vi "4060_outputs.vi"(0 "Address":T1, 3 "Value to Output":dbl format="%.2f", 4 "Channel Name":string) -> (5 "Comment":string, 6 "Reading":dbl format="%.3f")   [LabVIEW 2018]
uses:
  ADAM Client/Sub VIs/ADAM Controls/Address.ctl
panel:
  out "Digital output state byte":u8 format="%.0b"
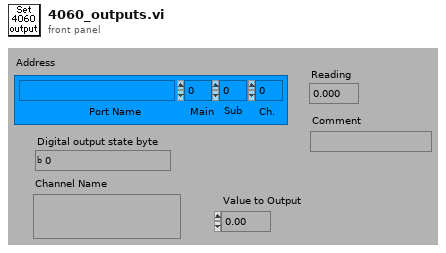
[diagram p1: front panel]
types:
  T1 = typedef "Address.ctl" = cluster{"Main":i32, "Ch.":i32, "Sub":i32, "Port Name":string}
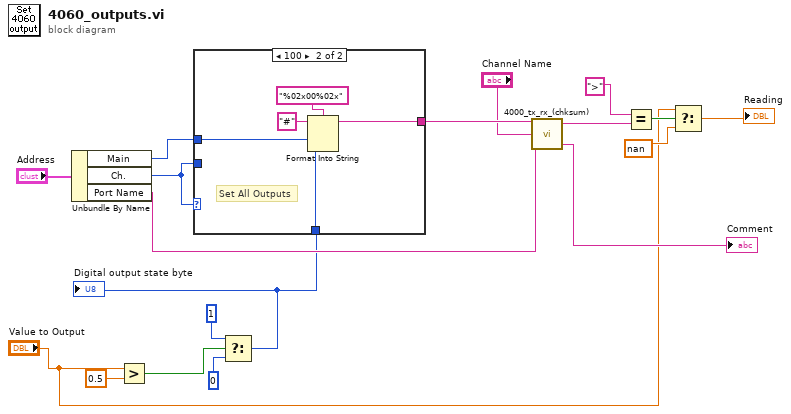
[diagram p0: block diagram]
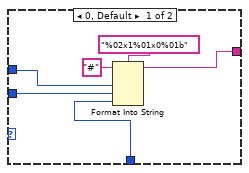
[diagram p2: hidden frame]
diagram:
  n1 = Unbundle By Name("Address") -> ("Main"=w9:i32, "Ch."=w8:i32, "Port Name"=w7:string)
  n2 = Greater?(x="Value to Output", y=0.5) -> (0:w3:bool)
  n3 = Select(t=u8 1 ("Digital output state byte"), s=w3, f=u8 0 ("Digital output state byte")) -> (s? t:f=w2:u8)
  "Digital output state byte" <- w2
  n4 = case shown="100" w8 {
    tunnel: w2 -> [w22 w29]
    tunnel: w9 -> [w20 w28]
    tunnel: [w19 w25] -> w18
    tunnel: w8 -> [w21 _]
    frame 0, Default {
      n5 = Format Into String(format string="%02x1%01x0%01b", initial string="#", w20, w21, w22) -> (resulting string=w19:string)  [unwired: 1 in, 1 out]
    }
    frame 100 {
      # "Set All Outputs"
      n6 = Format Into String(format string="%02x00%02x", initial string="#", w28, w29) -> (resulting string=w25:string)  [unwired: 1 in, 1 out]
    }
  }
  n7 = call "4000_tx_rx_(chksum).vi"("Write String"=w18, "Channel Name"="Channel Name", "Port Name"=w7) -> ("Read"=w15:string, "Comment out"=→"Comment":string)  [unwired: 2 in, 1 out]
  n8 = Equal?(x=">", y=w15) -> (x = y?=w13:bool)
  n9 = Select(t="Value to Output", s=w13, f=nan ("Reading")) -> (s? t:f=→"Reading":dbl)
